vi "Measure Simu.vi"(0 "OnOff.ACT":bool, 1 "ErrorAcknowledge.ACT":bool, 2 "Iteration Interval (s)":dbl, 3 "Channels In":T2(array[cluster]), 6 "Current Feedback In":dbl[](array[numeric]), 7 "Voltage Feedback In":dbl[](array[numeric]), 10 "Power Feedback In":dbl[](array[numeric]), 11 "Error Feedback In":bool[](array[boolean])) -> (8 "Current Feedback Out":dbl[](array[numeric]), 9 "Voltage Feedback Out":dbl[](array[numeric]), 12 "Power Feedback out":dbl[](array[numeric]), 13 "Error Feedback Out":bool[](array[boolean]), 14 "Channels Out":T1[](array[typedef]), 15 "Error Out":bool[](array[boolean]))   [LabVIEW 2023]
uses:
  C:/Program Files/National Instruments/AMS plugin/Capabilities/Capabilities/High Level Capabilities/Power Supply Cluster/Producer Ch.ctl
  C:/Program Files/National Instruments/AMS plugin/Capabilities/Capabilities/High Level Capabilities/Power Supply Cluster/Power Supply Cluster.lvclass
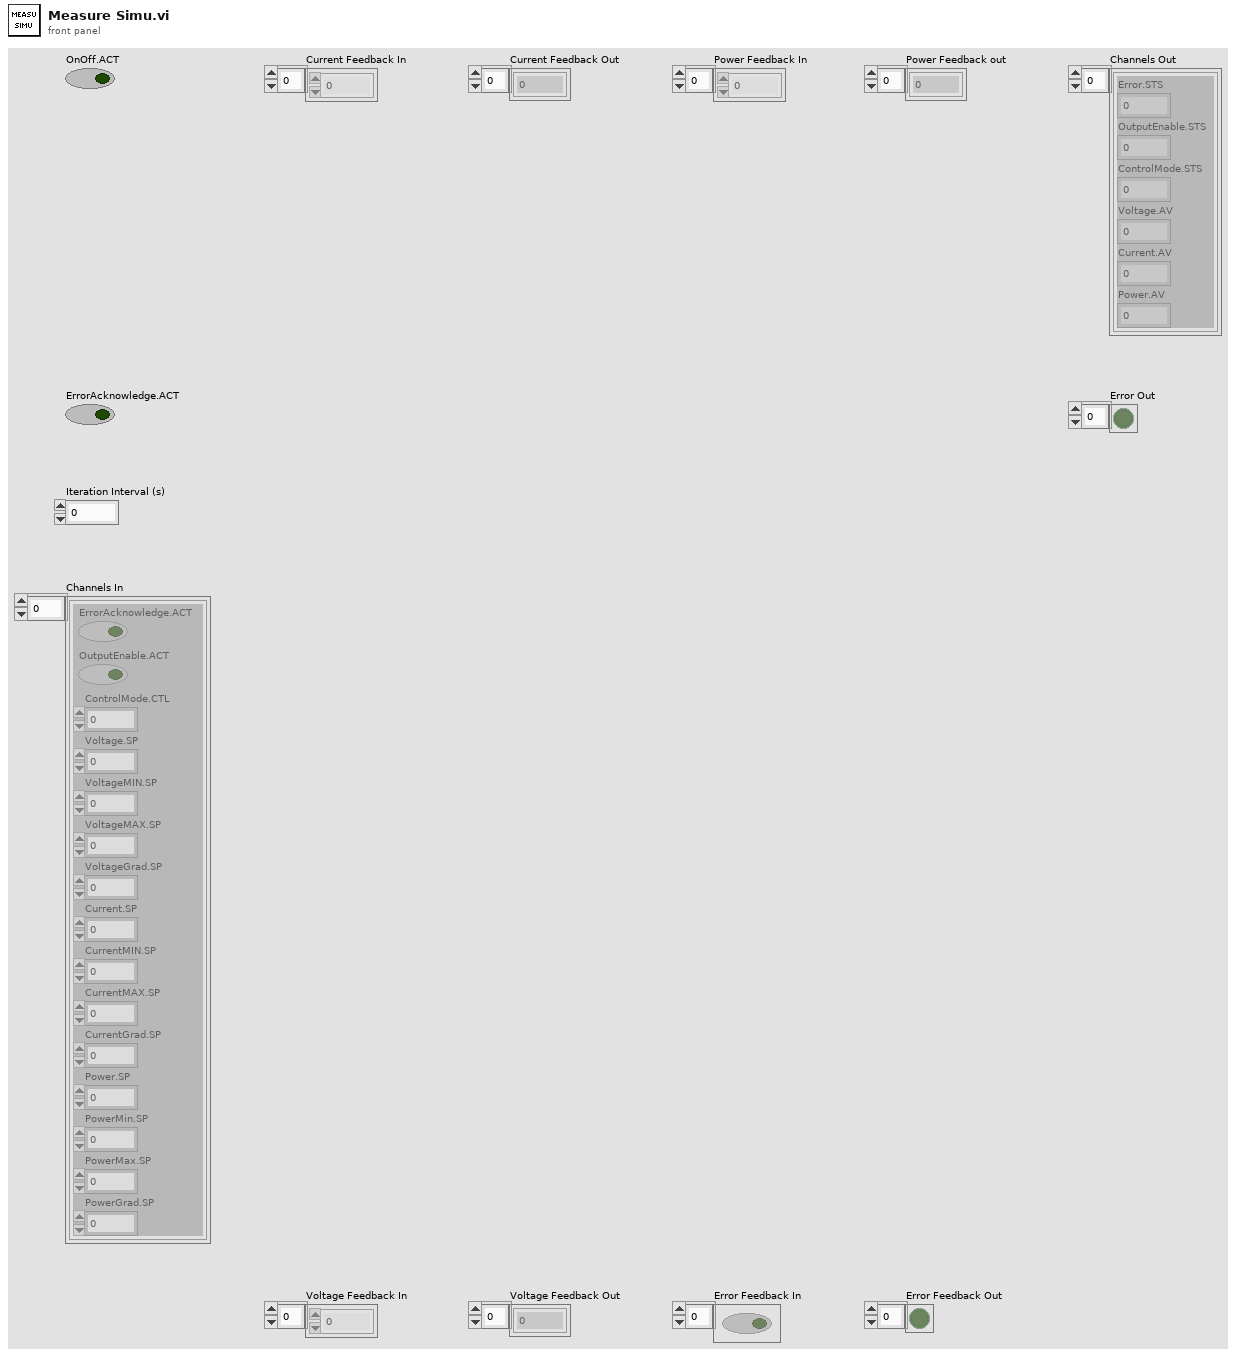
[diagram p1: front panel]
types:
  T1 = typedef "Power Supply Cluster.lvclass/Producer Ch.ctl" = cluster{"Error.STS":i32, "OutputEnable.STS":i32, "ControlMode.STS":u16, "Voltage.AV":dbl, "Current.AV":dbl, "Power.AV":dbl}
  T2 = cluster{"ErrorAcknowledge.ACT":bool, "OutputEnable.ACT":bool, "ControlMode.CTL":u16, "Voltage.SP":dbl, "VoltageMIN.SP":dbl, "VoltageMAX.SP":dbl, "VoltageGrad.SP":dbl, "Current.SP":dbl, "CurrentMIN.SP":dbl, "CurrentMAX.SP":dbl, "CurrentGrad.SP":dbl, "Power.SP":dbl, "PowerMin.SP":dbl, "PowerMax.SP":dbl, "PowerGrad.SP":dbl}[]
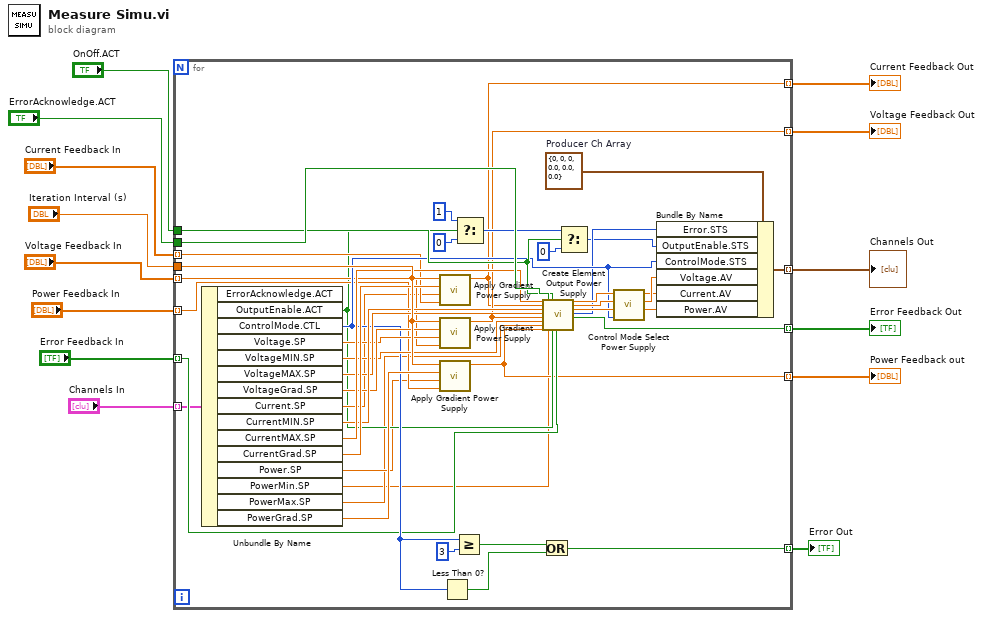
[diagram p0: block diagram]
diagram:
  n1 = for {
    tunnel: "ErrorAcknowledge.ACT" -> [w55]
    tunnel: "OnOff.ACT" -> [w54]
    tunnel: "Iteration Interval (s)" -> [w53]
    tunnel: "Channels In" -> [w28] mode=indexing
    tunnel: [w41] -> w2 mode=indexing
    tunnel: [w35] -> w5 mode=indexing
    tunnel: "Voltage Feedback In" -> [w34] mode=indexing
    tunnel: "Current Feedback In" -> [w33] mode=indexing
    tunnel: [w29] -> w6 mode=indexing
    tunnel: "Power Feedback In" -> [w32] mode=indexing
    tunnel: [w17] -> w4 mode=indexing
    tunnel: [w21] -> w3 mode=indexing
    tunnel: "Error Feedback In" -> [w31] mode=indexing
    tunnel: [w22] -> w1 mode=indexing
    w15 = T1 {"Error.STS"=0, "OutputEnable.STS"=0, "ControlMode.STS"=0, "Voltage.AV"=0.0, "Current.AV"=0.0, "Power.AV"=0.0}  # Producer Ch Array
    n2 = Unbundle By Name(w28) -> ("OutputEnable.ACT"=w20:bool, "ControlMode.CTL"=w36:u16, "Voltage.SP"=w45:dbl, "VoltageMIN.SP"=w46:dbl, "VoltageMAX.SP"=w47:dbl, "VoltageGrad.SP"=w48:dbl, "Current.SP"=w30:dbl, "CurrentMIN.SP"=w49:dbl, "CurrentMAX.SP"=w50:dbl, "CurrentGrad.SP"=w51:dbl, "Power.SP"=w19:dbl, "PowerMin.SP"=w16:dbl, "PowerMax.SP"=w18:dbl, "PowerGrad.SP"=w52:dbl)  [unwired: 1 out]
    n3 = call "Apply Gradient Power Supply.vi"("Reminder"=w33, "Setpoint"=w30, "Gradient"=w51, "Iteration Interval"=w53) -> ("Current Setpoint"=w29:dbl)  [unwired: 7 in]
    n4 = call "Apply Gradient Power Supply.vi"("Reminder"=w34, "Setpoint"=w45, "Gradient"=w48, "Iteration Interval"=w53) -> ("Current Setpoint"=w35:dbl)  [unwired: 7 in]
    n5 = call "Apply Gradient Power Supply.vi"("Reminder"=w32, "Setpoint"=w19, "Gradient"=w52, "Iteration Interval"=w53) -> ("Current Setpoint"=w17:dbl)  [unwired: 7 in]
    n6 = Less Than 0?(x=w36) -> (x < 0?=w43:bool)
    n7 = Greater Or Equal?(x=w36, y=u16 3) -> (x >= y?=w44:bool)
    n8 = Select(t=1, s=w20, f=0) -> (s? t:f=w37:i32)
    n9 = Or(x=w44, y=w43) -> (x .or. y?=w41:bool)
    n10 = call "Create Element Output Power Supply.vi"("Current Max SP"=w50, "Current In"=w29, "Current Min SP"=w49, "Voltage Max SP"=w47, "Voltage In"=w35, "Voltage Min SP"=w46, "Power Max SP"=w18, "Power In"=w17, "Error ACT"=w55, "Power Min SP"=w16, "OnOff ACT"=w54, "Output Enable ACT"=w20, "Feedback In"=w31) -> ("Current Out"=w58:dbl, "Voltage Out"=w57:dbl, "Power Out"=w56:dbl, "Error Channels"=w27:i32, "Feedback Out"=w21:bool)  [unwired: 10 in]
    n11 = Select(t=w37, s=w54, f=0) -> (s? t:f=w26:i32)
    n12 = call "Control Mode Select Power Supply.vi"("Control Mode Read"=w36, "Power Read"=w56, "Voltage Read"=w57, "Current Read"=w58) -> ("Power Write"=w23:dbl, "Voltage Write"=w25:dbl, "Current Write"=w24:dbl)  [unwired: 5 in]
    n13 = Bundle By Name(cluster=w15, "Error.STS"=w27, "OutputEnable.STS"=w26, "ControlMode.STS"=w36, "Voltage.AV"=w25, "Current.AV"=w24, "Power.AV"=w23) -> (w22:T1)
  }
  "Current Feedback Out" <- w6
  "Voltage Feedback Out" <- w5
  "Power Feedback out" <- w4
  "Error Feedback Out" <- w3
  "Error Out" <- w2
  "Channels Out" <- w1
